vi "WriteArrData.vi"(6 "IndPoint":i32, 8 "error in (no error)":errorcluster caption="entrée d'erreur (pas d'erreur)", 11 "Interface en entrée":refnum<class "Interface.lvclass"> caption="DNL_LabVIEW Object in") -> (0 "error out":errorcluster caption="sortie d'erreur", 1 "CrvIndex":i32, 2 "CurCrvPointInd":i32, 3 "Interface en sortie":refnum<class "Interface.lvclass"> caption="DNL_LabVIEW Object out")   [LabVIEW 2019, in "Interface.lvclass"]
uses:
  Interface.lvclass
  Experiment Class/Experiment.lvclass
  Interface.lvclass/Interface.ctl
  DevicesClass/BaseDevice/BaseDevice.lvclass
panel:
  in  "ArrayDevData":cluster{"DevIndex":i32, "MeasDatOut":dbl[][]}[](array[cluster])
  in  "Experiment.lvclass In":refnum<class "Experiment.lvclass">
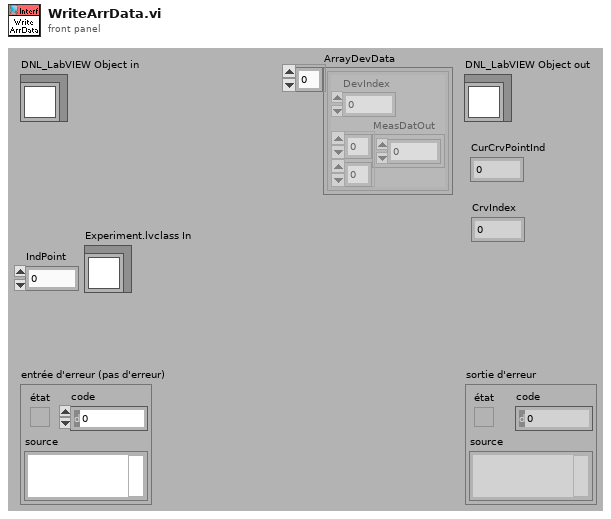
[diagram p1: front panel]
types:
  T1 = enum16{"open", "replace", "create", "open or create", "replace or create", "replace or create with confirmation"}
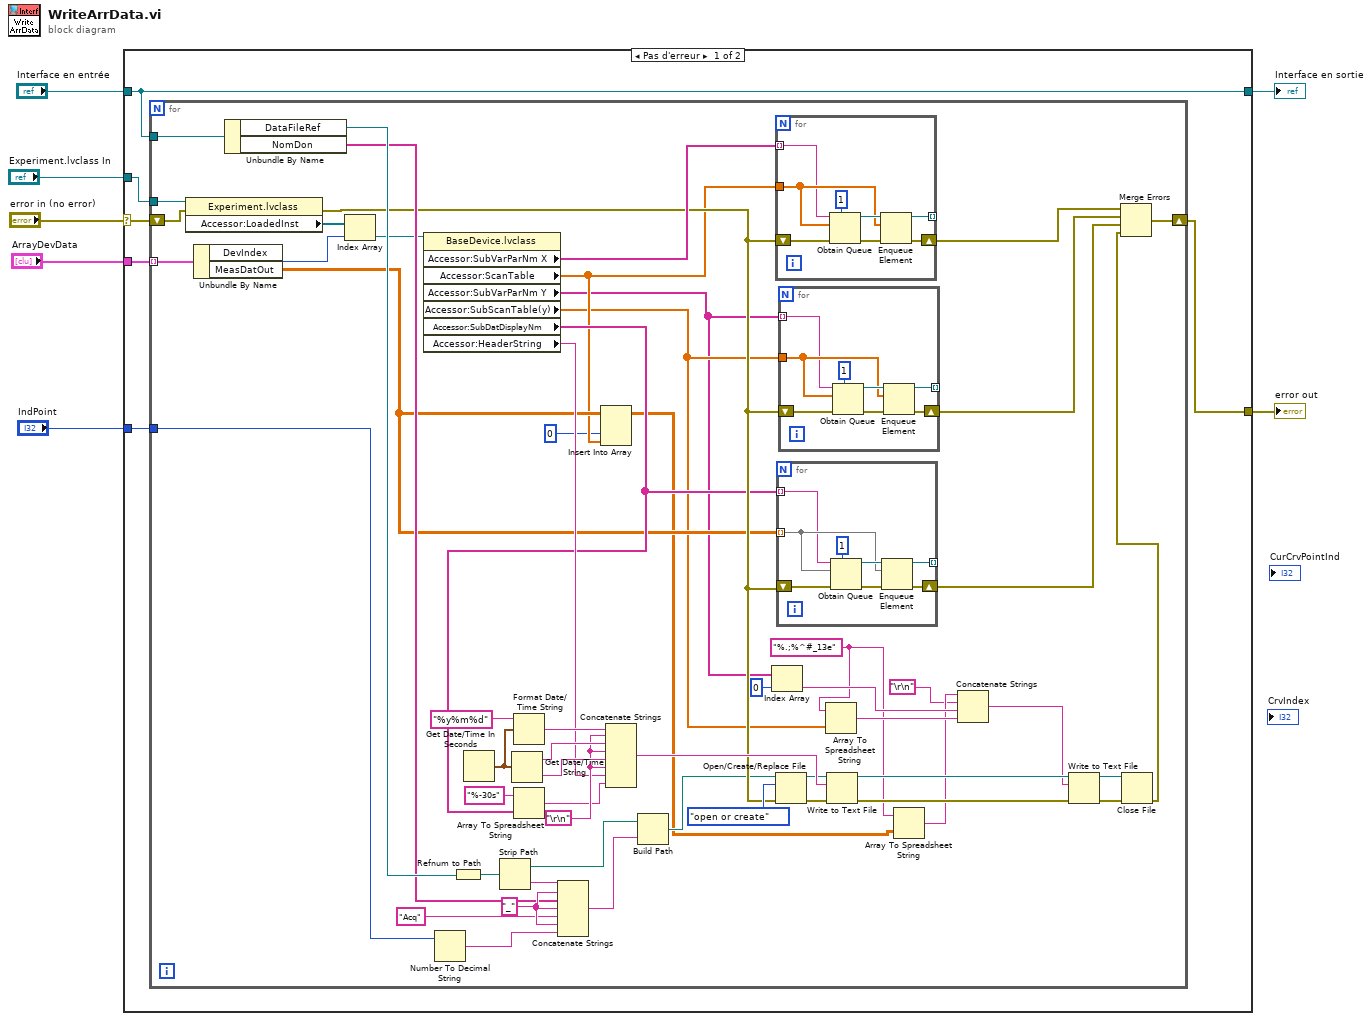
[diagram p0: block diagram]
diagram:
  n1 = case shown="Pas d'erreur" "error in (no error)" {
    selector: "error in (no error)" -> [w9 w95]
    tunnel: [w8 w95] -> w6
    tunnel: [w12 w94] -> w4
    tunnel: "Interface en entrée" -> [w12 w94]
    tunnel: "IndPoint" -> [w13 _]
    tunnel: "Experiment.lvclass In" -> [w11 _]
    tunnel: "ArrayDevData" -> [w10 _]
    frame No Error {
      n2 = for {
        tunnel: w13 -> [w63]
        tunnel: w12 -> [w62]
        tunnel: w11 -> [w58]
        tunnel: w10 -> [w55] mode=indexing
        shift-right: [w22] -> w8
        shift-left: w9 -> [w57]
        w17 = "%.;%^#_13e" ("chaîne de format")
        w44 = "\r\n"
        w67 = "_" ("chaîne")
        n3 = property class="Experiment.lvclass"(reference=w58, error in=w57) -> (error out=w41:errorcluster, "Accessor:LoadedInst"=w56:refnum<class "BaseDevice.lvclass">[])  [unwired: 1 out]
        n4 = Unbundle By Name(w55) -> ("DevIndex"=w54:i32, "MeasDatOut"=w34:dbl[][])
        n5 = Unbundle By Name(w62) -> ("DataFileRef"=w61:refnum<file>, "NomDon"=w60:string[])
        n6 = Index Array(array=w56, index=w54) -> (element=w53:refnum<class "BaseDevice.lvclass">)
        n7 = property class="BaseDevice.lvclass"(reference=w53) -> ("Accessor:SubVarParNm X"=w52:string[], "Accessor:ScanTable"=w33:dbl[], "Accessor:SubVarParNm Y"=w28:string[], "Accessor:SubScanTable(y)"=w30:dbl[], "Accessor:SubDatDisplayNm"=w37:string[], "Accessor:HeaderString"=w43:string)  [unwired: 1 in, 2 out]
        n8 = Number To Decimal String(number=w63) -> (decimal integer string=w66:string)  [unwired: 1 in]
        n9 = Refnum to Path(1:w61) -> (0:w69:path)
        n10 = Get Date/Time In Seconds() -> (seconds since 1Jan1904=w50:timestamp)
        n11 = Strip Path(path=w69) -> (stripped path=w65:path, name=w68:string)
        n12 = Get Date/Time String(seconds (now)=w50) -> (date string=w46:string, time string=w45:string)  [unwired: 2 in]
        n13 = Format Date/Time String(time format string (%c)="%y%m%d" ("chaîne de format de l'heure (%c)"), seconds (now)=w50) -> (date/time string=w47:string)  [unwired: 1 in]
        n14 = Array To Spreadsheet String(array=w37, 3:"%-30s" ("chaîne de format")) -> (spreadsheet string=w35:string)  [unwired: 1 in]
        n15 = Concatenate Strings(w68, w67, w60, w67, "Acq" ("chaîne"), w67, w66) -> (w64:string)
        n16 = Insert Into Array(array=w34, index (col)=0 ("indice désactivé (col)"), new element=w33) -> (w16:dbl[][])  [unwired: 1 in]
        n17 = Concatenate Strings(w47, w44, w46, w44, w45, w44, w43, w35) -> (w42:string)
        n18 = Build Path(base path=w65, name or relative path=w64) -> (appended path=w31:path)
        n19 = Index Array(array=w28, index=0 ("indice")) -> (element=w26:string)
        n20 = for {
          tunnel: [w90] -> _ mode=indexing
          tunnel: w33 -> [w89]
          shift-right: [w91] -> w21
          shift-left: w41 -> [w88]
          tunnel: w52 -> [w87] mode=indexing
          n21 = Obtain Queue(max queue size (-1, unlimited)=1 ("taille max de la file d'attente (-1, non limitée)"), name (unnamed)=w87, element data type=w89, error in (no error)=w88) -> (queue out=w92:refnum<queue>, error out=w93:errorcluster)  [unwired: 1 in, 1 out]
          n22 = Enqueue Element(queue=w92, element=w89, error in (no error)=w93) -> (queue out=w90:refnum<queue>, error out=w91:errorcluster)  [unwired: 1 in, 1 out]
        }
        n23 = Open/Create/Replace File(file path (use dialog)=w31, error in=w41, operation (0:open)=T1."open or create" ("opération (0 : open)")) -> (refnum out=w39:refnum<file>, error out=w40:errorcluster)  [unwired: 3 in, 1 out]
        n24 = for {
          tunnel: [w82] -> _ mode=indexing
          tunnel: w34 -> [w81] mode=indexing
          shift-right: [w83] -> w19
          shift-left: w41 -> [w80]
          tunnel: w37 -> [w79] mode=indexing
          n25 = Obtain Queue(max queue size (-1, unlimited)=1 ("taille max de la file d'attente (-1, non limitée)"), name (unnamed)=w79, element data type=w81, error in (no error)=w80) -> (queue out=w84:refnum<queue>, error out=w85:errorcluster)  [unwired: 1 in, 1 out]
          n26 = Enqueue Element(queue=w84, element=w81, error in (no error)=w85) -> (queue out=w82:refnum<queue>, error out=w83:errorcluster)  [unwired: 1 in, 1 out]
        }
        n27 = for {
          tunnel: [w74] -> _ mode=indexing
          tunnel: w30 -> [w73]
          shift-right: [w75] -> w20
          shift-left: w41 -> [w72]
          tunnel: w28 -> [w71] mode=indexing
          n28 = Obtain Queue(max queue size (-1, unlimited)=1 ("taille max de la file d'attente (-1, non limitée)"), name (unnamed)=w71, element data type=w73, error in (no error)=w72) -> (queue out=w76:refnum<queue>, error out=w77:errorcluster)  [unwired: 1 in, 1 out]
          n29 = Enqueue Element(queue=w76, element=w73, error in (no error)=w77) -> (queue out=w74:refnum<queue>, error out=w75:errorcluster)  [unwired: 1 in, 1 out]
        }
        n30 = Array To Spreadsheet String(array=w30, 3:w17) -> (spreadsheet string=w29:string)  [unwired: 1 in]
        n31 = Write to Text File(file (use dialog)=w39, text=w42, error in=w40) -> (refnum out=w51:refnum<file>, error out=w38:errorcluster)  [unwired: 1 in, 1 out]
        n32 = Array To Spreadsheet String(array=w16, 3:w17) -> (spreadsheet string=w15:string)  [unwired: 1 in]
        n33 = Concatenate Strings(w15, "\r\n", w26, w29) -> (w25:string)
        n34 = Write to Text File(file (use dialog)=w51, text=w25, error in=w38) -> (refnum out=w23:refnum<file>, error out=w24:errorcluster)  [unwired: 1 in, 1 out]
        n35 = Close File(refnum=w23, error in=w24) -> (error out=w18:errorcluster)  [unwired: 1 out]
        n36 = Merge Errors(w21, w20, w19, w18) -> (w22:errorcluster)
      }
    }
    frame Error {
    }
  }
  "error out" <- w6
  "Interface en sortie" <- w4
